vi "myDAQ 2AnalogSensors_DAQAssistant.vi"() -> ()   [LabVIEW 2018]
uses:
  <vilib>/express/express analysis/Spectral/Block/exnSpectralBlock spectral measurements power poly.vi
  <vilib>/express/express analysis/Spectral/Block/exnSpectralBlock spectral measurements power DDT.vi
  <vilib>/express/express analysis/Spectral/XNode/ExpressSpectralMeasurementsBlockNode.xnode
panel:
  out "return value":string
  in  "module path":path
  out "Frequency Max":dbl
  out "Amplitude Max":dbl
  out "Power Spectrum":dynamicdata(graph)
  out "Wave\nRepresentation":dynamicdata(graph)
  out "data":dynamicdata(graph)
  in  "stop (F)":bool
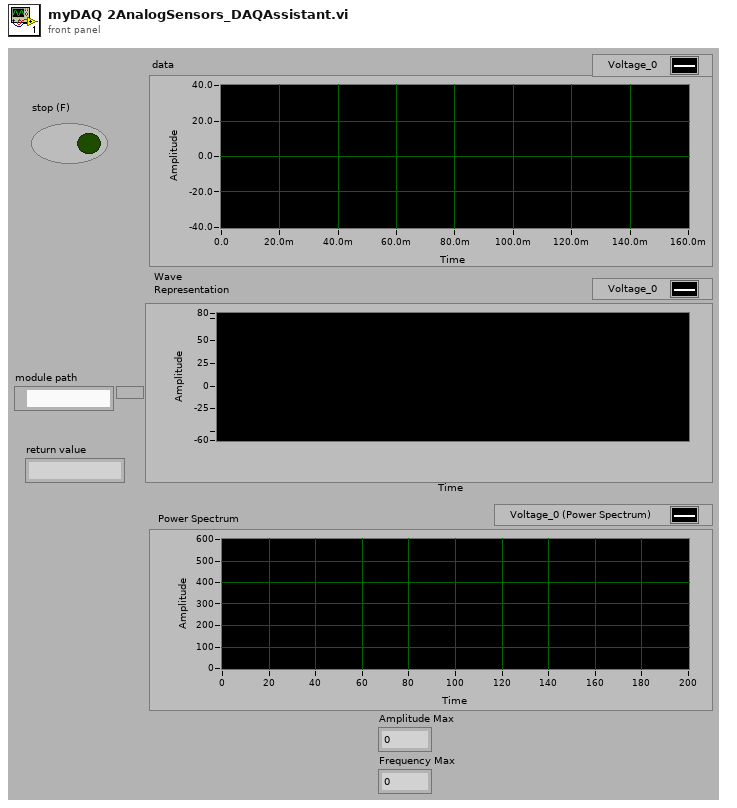
[diagram p1: front panel]
types:
  T1 = cluster{"averaging mode":u16, "weighting mode":u16, "number of averages":u32}
  T2 = cluster{"dB On (F)":bool, "unwrap phase (F)":bool, "convert to degree (F)":bool}
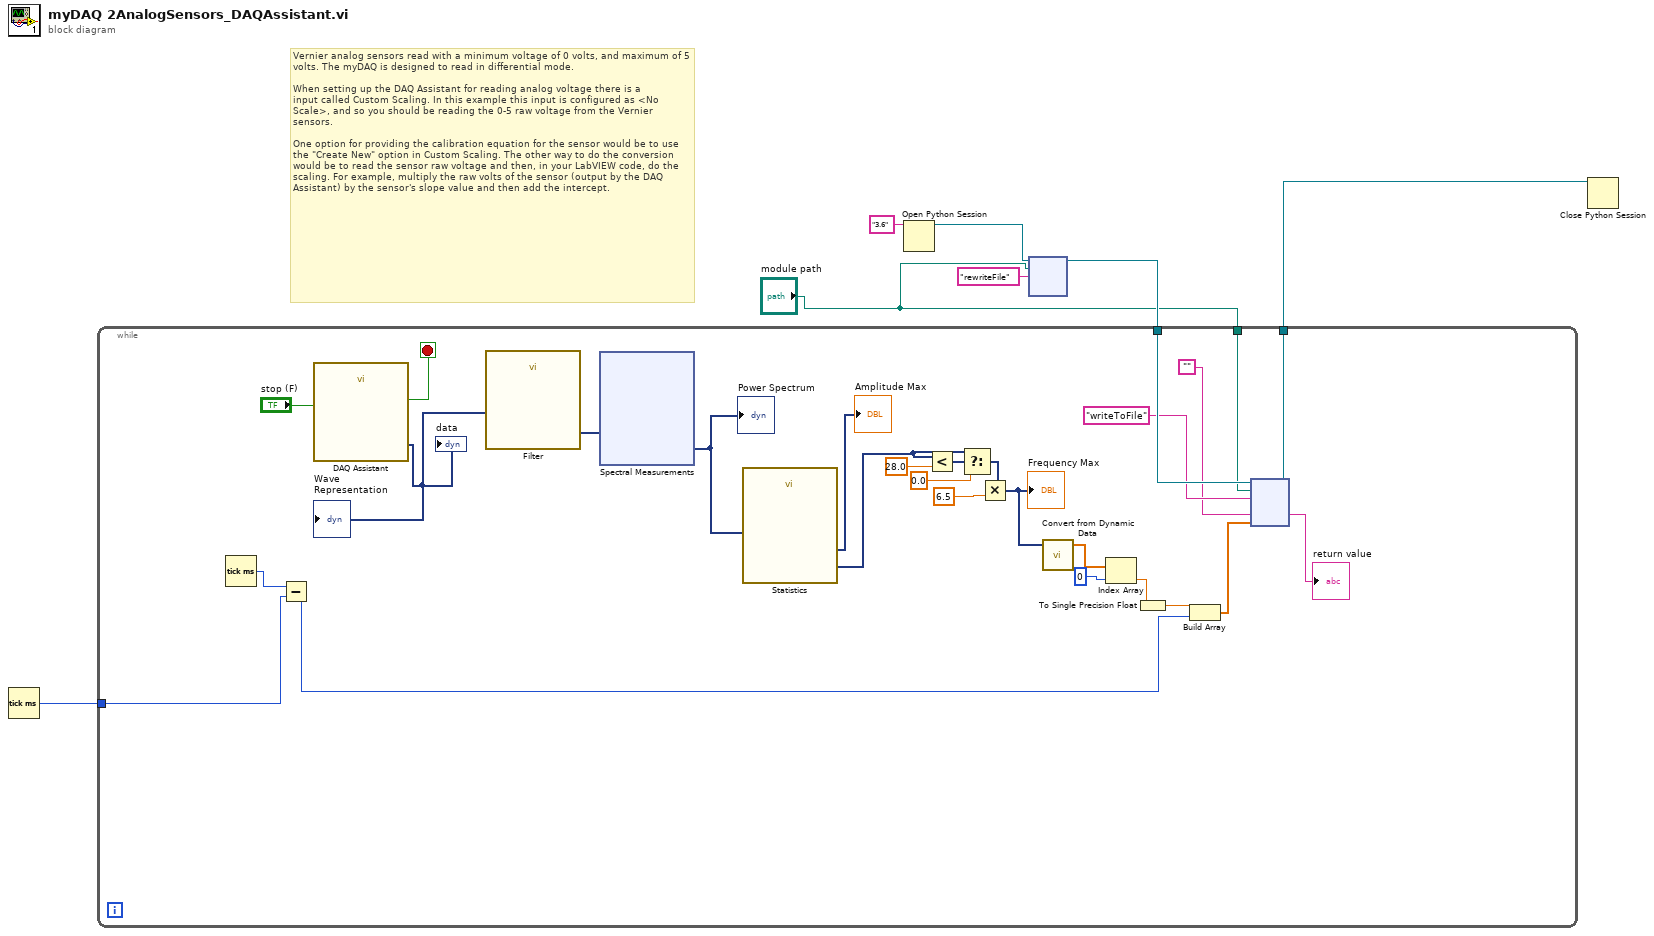
[diagram p0: block diagram]
diagram:
  # "Vernier analog sensors read with a minimum voltage of 0 volts, and maximum of 5 volts. The myDAQ is designed to read in differential mode.\n\nWhen setting up the DAQ Assistant for reading analog voltage there is a \ninput called Custom Scaling. In this example this input is configured as <No Scale>, and so you should be reading the 0-5 raw voltage from the Vernier sensors. \n\nOne option for providing the calibration equation for the sensor would be to use the \"Create New\" option in Custom Scaling. The other way to do the conversion would be to read the sensor raw voltage and then, in your LabVIEW code, do the scaling. For example, multiply the raw volts of the sensor (output by the DAQ Assistant) by the sensor's slope value and then add the intercept."
  n1 = Tick Count (ms)() -> (millisecond timer value=w6:u32)
  n2 = Open Python Session(python version="3.6" ("Python version")) -> (session out=w4:refnum<k35>)  [unwired: 2 in, 1 out]
  n3 = node(w4, "module path", "rewriteFile" ("function name")) -> (w3:refnum<k35>)  [unwired: 3 in, 3 out]
  n4 = while {
    tunnel: w3 -> [w21]
    tunnel: [w20] -> w1
    tunnel: "module path" -> [w19]
    tunnel: w6 -> [w14]
    stop <- w33 stop-if-true
    n5 = Tick Count (ms)() -> (millisecond timer value=w22:u32)
    n6 = Subtract(x=w22, y=w14) -> (x-y=w13:u32)
    n7 = call "DAQ Assistant"("stop (F)"="stop (F)") -> ("data"=w32:dynamicdata, "stopped"=w33:bool)  [unwired: 15 in, 2 out]
    "data" <- w32
    "Wave\nRepresentation" <- w32
    n8 = call "Filter"("Signal"=w32) -> ("Filtered Signal"=w31:dynamicdata)  [unwired: 9 in, 1 out]
    n9 = xnode "Spectral Measurements"("Signals"=w31) -> ("Power Spectrum"=w29:dynamicdata)  [unwired: 1 in, 1 out]
    "Power Spectrum" <- w29
    n10 = call "Statistics"("Signals"=w29) -> ("Index of Max"=w26:dynamicdata, "Maximum"=→"Amplitude Max":dynamicdata)  [unwired: 24 in, 1 out]
    n11 = Less?(x=w26, y=28.0) -> (x < y?=w27:dynamicdata)
    n12 = Select(t=w26, s=w27, f=0.0) -> (s? t:f=w23:dynamicdata)
    n13 = Multiply(x=w23, y=6.5) -> (x*y=w18:dynamicdata)
    "Frequency Max" <- w18
    n14 = call "Convert from Dynamic Data"("Dynamic Data Type"=w18) -> ("Array"=w16:dbl[])  [unwired: 3 in]
    n15 = Index Array(array=w16, index=0) -> (element=w11:dbl)
    n16 = To Single Precision Float(number=w11) -> (single precision float=w10:sgl)
    n17 = Build Array(w10, w13) -> (w12:sgl[])
    n18 = node(w21, w19, "writeToFile" ("function name"), "", w12) -> (w20:refnum<k35>, →"return value":string)  [unwired: 2 in, 3 out]
  }
  n19 = Close Python Session(session in=w1) -> ()  [unwired: 1 in, 1 out]
